vi "emi_Create Cluster Variant.vi"(0 "Cluster":variant, 5 "Cluster Elements":variant[](array[variant]), 11 "error in (no error)":errorcluster) -> (4 "Cluster Out":variant, 15 "error out":errorcluster)   [LabVIEW 2011]
doc: "Connect a variant of an cluster, and an array of variants of the Cluster elements, containing the values.\nReturned is a variant holding the cluster with values.\n\nMade as a replace ment for the SetClusterInfo.vi from NI, which should be doing this.\nThe array of Variants can be gotten from the NI vi: GetClusterInfo.vi\n\nIntende use: Ini file. May be extended to other reading and writing of cluster data\n\nOn Error:No Action"
uses:
  Error/emi_Create Error.vi
  <vilib>/Utility/VariantDataType/GetNumericInfo.vi
  <vilib>/Utility/VariantDataType/VariantType.lvlib
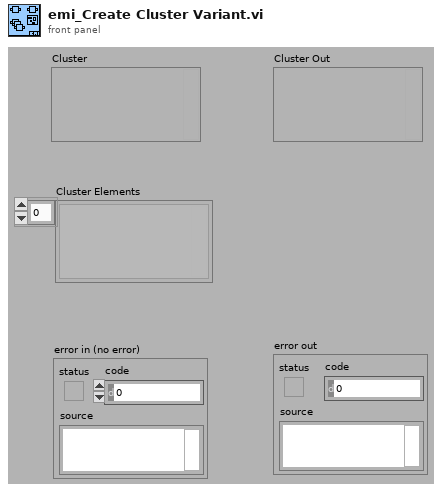
[diagram p1: front panel]
types:
  T1 = typedef "VariantType.lvlib/Type.ctl" = enum8{"Invalid Type", "Void", "I8", "I16", "I32", "I64", "U8", "U16", "U32", "U64", "Single Float", "Double Float", "Extended Float", "Single Complex", "Double Complex", "Extended Complex", "Enum U8", "Enum U16", "Enum U32", "Enum U64", "Single Float With Unit", "Double Float With Unit", "Extended Float With Unit", "Single Complex with Unit", "Double Complex with Unit", "Extended Complex with Unit", "Boolean", "String", "Path", "Picture", "Tag", "Array", "Cluster", "Variant", "LV Variant", "Waveform", "Timestamp", "Digital Waveform", "Digital Data", "ExpressData", "Refnum", "External Data", "VI", "Poly VI", "LabVIEW Class Instance", "Fixed Point"}
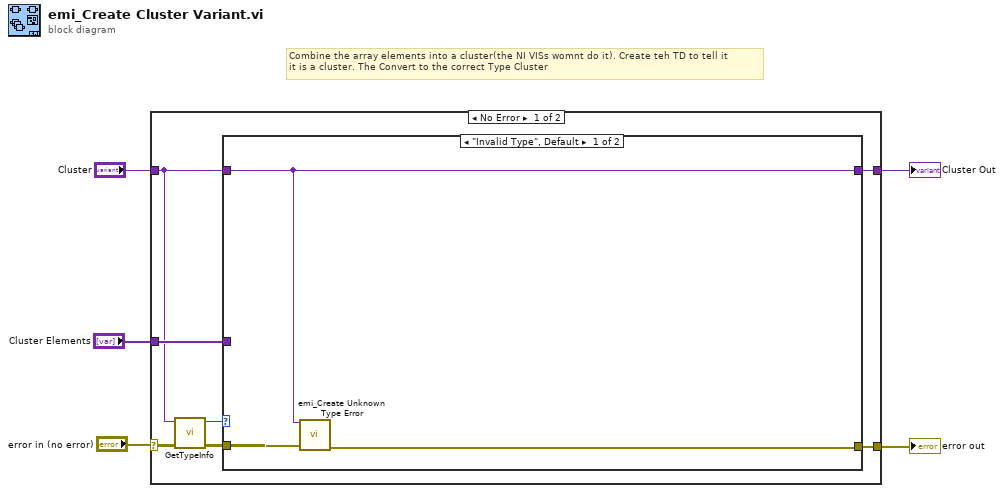
[diagram p0: block diagram]
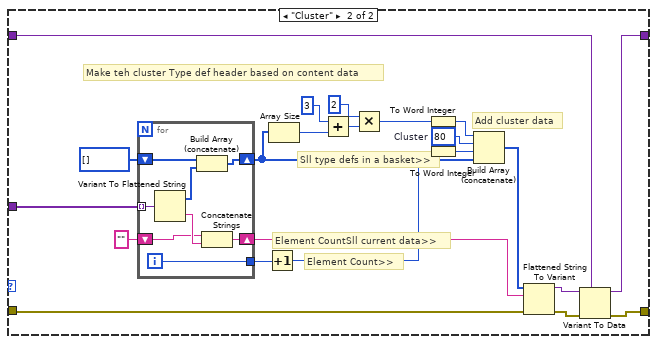
[diagram p2: hidden frame]
diagram:
  # "Combine the array elements into a cluster(the NI VISs womnt do it). Create teh TD to tell it\nit is a cluster. The Convert to the correct Type Cluster"
  n1 = case shown="No Error" "error in (no error)" {
    selector: "error in (no error)" -> [w9 w46]
    tunnel: "Cluster Elements" -> [w12 _]
    tunnel: [w11 w47] -> w4
    tunnel: [w10 w46] -> w3
    tunnel: "Cluster" -> [w7 w47]
    frame No Error {
      n2 = call <vilib>:"GetTypeInfo.vi"("error in (no error)"=w9, "Variant"=w7) -> ("error out"=w8:errorcluster, "Type Enum"=w6:T1)  [unwired: 5 in, 3 out]
      n3 = case shown="\"Invalid Type\", Default" w6 {
        tunnel: w12 -> [_ w22]
        tunnel: [w13 w21] -> w11
        tunnel: [w14 w20] -> w10
        tunnel: w8 -> [w15 w17]
        tunnel: w7 -> [w13 w16]
        frame "Invalid Type", Default {
          n4 = call "emi_Create Unknown Type Error.vi"("Anything"=w13, "error IO"=w15) -> ("error out"=w14:errorcluster)  [unwired: 13 in]
        }
        frame "Cluster" {
          w30 = i16 80  # Cluster
          # "Add cluster data"
          # "Make teh cluster Type def header based on content data"
          # "Element CountSll current data>>"
          # "Sll type defs in a basket>>"
          # "Element Count>>"
          n5 = for {
            tunnel: w22 -> [w45] mode=indexing
            shift-right: [w43] -> w34
            shift-left: i16[] [] -> [w42]
            tunnel: [w41] -> w24
            shift-right: [w39] -> w35
            shift-left: "" -> [w38]
            i -> [w41]
            n6 = Variant To Flattened String(Variant=w45) -> (data string=w40:string, 1:w44:i16[])
            n7 = Build Array (concatenate)(w42, w44) -> (w43:i16[])
            n8 = Concatenate Strings(w38, w40) -> (w39:string)
          }
          n9 = Increment(x=w24) -> (x+1=w33:i32)
          n10 = Array Size(array=w34) -> (size(s)=w25:i32)
          n11 = Add(x=3, y=w25) -> (x+y=w26:i32)
          n12 = Multiply(x=2, y=w26) -> (x*y=w29:i32)
          n13 = To Word Integer(number=w29) -> (16bit integer=w31:i16)
          n14 = To Word Integer(number=w33) -> (16bit integer=w32:i16)
          n15 = Build Array (concatenate)(w31, w30, w32, w34) -> (w36:i16[])
          n16 = Flattened String To Variant(4:w17, 6:w35, 7:w36) -> (0:w18:errorcluster, 3:w19:variant)
          n17 = Variant To Data(error in=w18, type=w16, Variant=w19) -> (data=w21:variant, error out=w20:errorcluster)
        }
      }
    }
    frame Error {
    }
  }
  "error out" <- w3
  "Cluster Out" <- w4
